vi "Measure Voltage.vi"(7 "Channel Lists":string[](array[string]), 8 "error in (no error)":errorcluster, 10 "Delay Time (s)":dbl, 11 "DCPower Sessions In":refnum<k15>[](array[refnum])) -> (0 "error out":errorcluster, 1 "Voltage measurements":dbl[][](array[numeric]), 3 "DCPower Sessions Out":refnum<k15>[](array[refnum]))   [LabVIEW 2013]
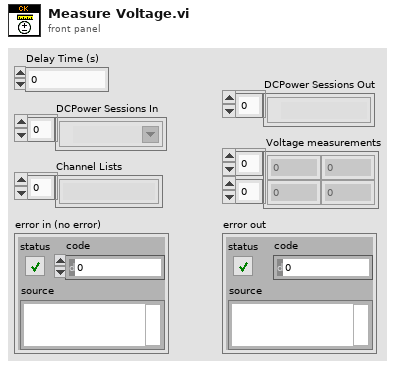
[diagram p1: front panel]
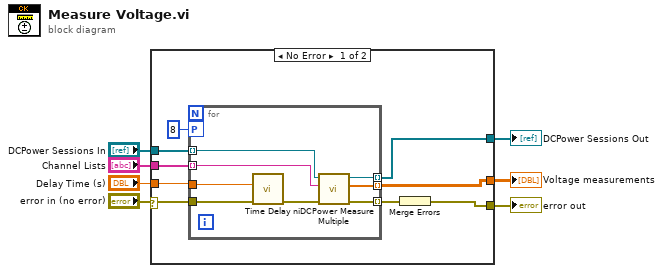
[diagram p0: block diagram]
diagram:
  n1 = case shown="No Error" "error in (no error)" {
    selector: "error in (no error)" -> [w10 w25]
    tunnel: "Channel Lists" -> [w16 _]
    tunnel: "DCPower Sessions In" -> [w15 w26]
    tunnel: [w14 w26] -> w5
    tunnel: [w12 w25] -> w4
    tunnel: "Delay Time (s)" -> [w11 _]
    tunnel: [w8 _] -> w2
    frame No Error {
      n2 = for {
        tunnel: w10 -> [w21]
        tunnel: w15 -> [w19] mode=indexing
        tunnel: w16 -> [w23] mode=indexing
        tunnel: [w24] -> w13 mode=indexing
        tunnel: [w17] -> w8 mode=indexing
        tunnel: [w22] -> w14 mode=indexing
        tunnel: w11 -> [w18]
        workers-P: 8 -> [_]
        n3 = call "Time Delay"("error in (no error)"=w21, "Delay Time (s)"=w18) -> ("error out"=w20:errorcluster)  [unwired: 9 in]
        n4 = call <instrlib>:"niDCPower Measure Multiple.vi"("error in (no error)"=w20, "channel name"=w23, "instrument handle"=w19) -> ("error out"=w24:errorcluster, "voltage measurements"=w17:dbl[], "instrument handle out"=w22:refnum<k15>)  [unwired: 5 in, 1 out]
      }
      n5 = Merge Errors(w13) -> (w12:errorcluster)
    }
    frame Error {
    }
  }
  "Voltage measurements" <- w2
  "DCPower Sessions Out" <- w5
  "error out" <- w4
